vi "Overview.vi"() -> ()   [LabVIEW 2017]
panel:
  out "Time":sgl format="%#_13g"
  out "Flow Rate":sgl caption="C" format="%.1f"
  out "TCHX Power":sgl caption="C" format="%.1f"
  out "DHX Power":dbl caption="C" format="%.1f"
  out "Thermal Power":sgl format="%.1f"
  out "Electrical Power":sgl format="%.1f"
  in  "stop":bool
  out "Fluid Min Temp":sgl format="%.1f"
  out "CTAH Power":sgl format="%.1f"
  out "Fluid Max Temp":sgl format="%.1f"
  out "Heater Power":sgl caption="C" format="%.1f"
  out "LPT Work":sgl format="%.1f"
  out "HPT Work":sgl format="%.1f"
  out "Compressor Work":sgl format="%.1f"
  out "Ambient Temperature":sgl format="%.1f"
  # "Overview"
  # "TCHX"
  # "LPT"
  # "HPT"
  # "COMPRESSOR"
  # "DHX"
  # "CTAH"
  # "HEATER"
  # "PUMP"
  # "NOAH Jr."
  # "Procedures"
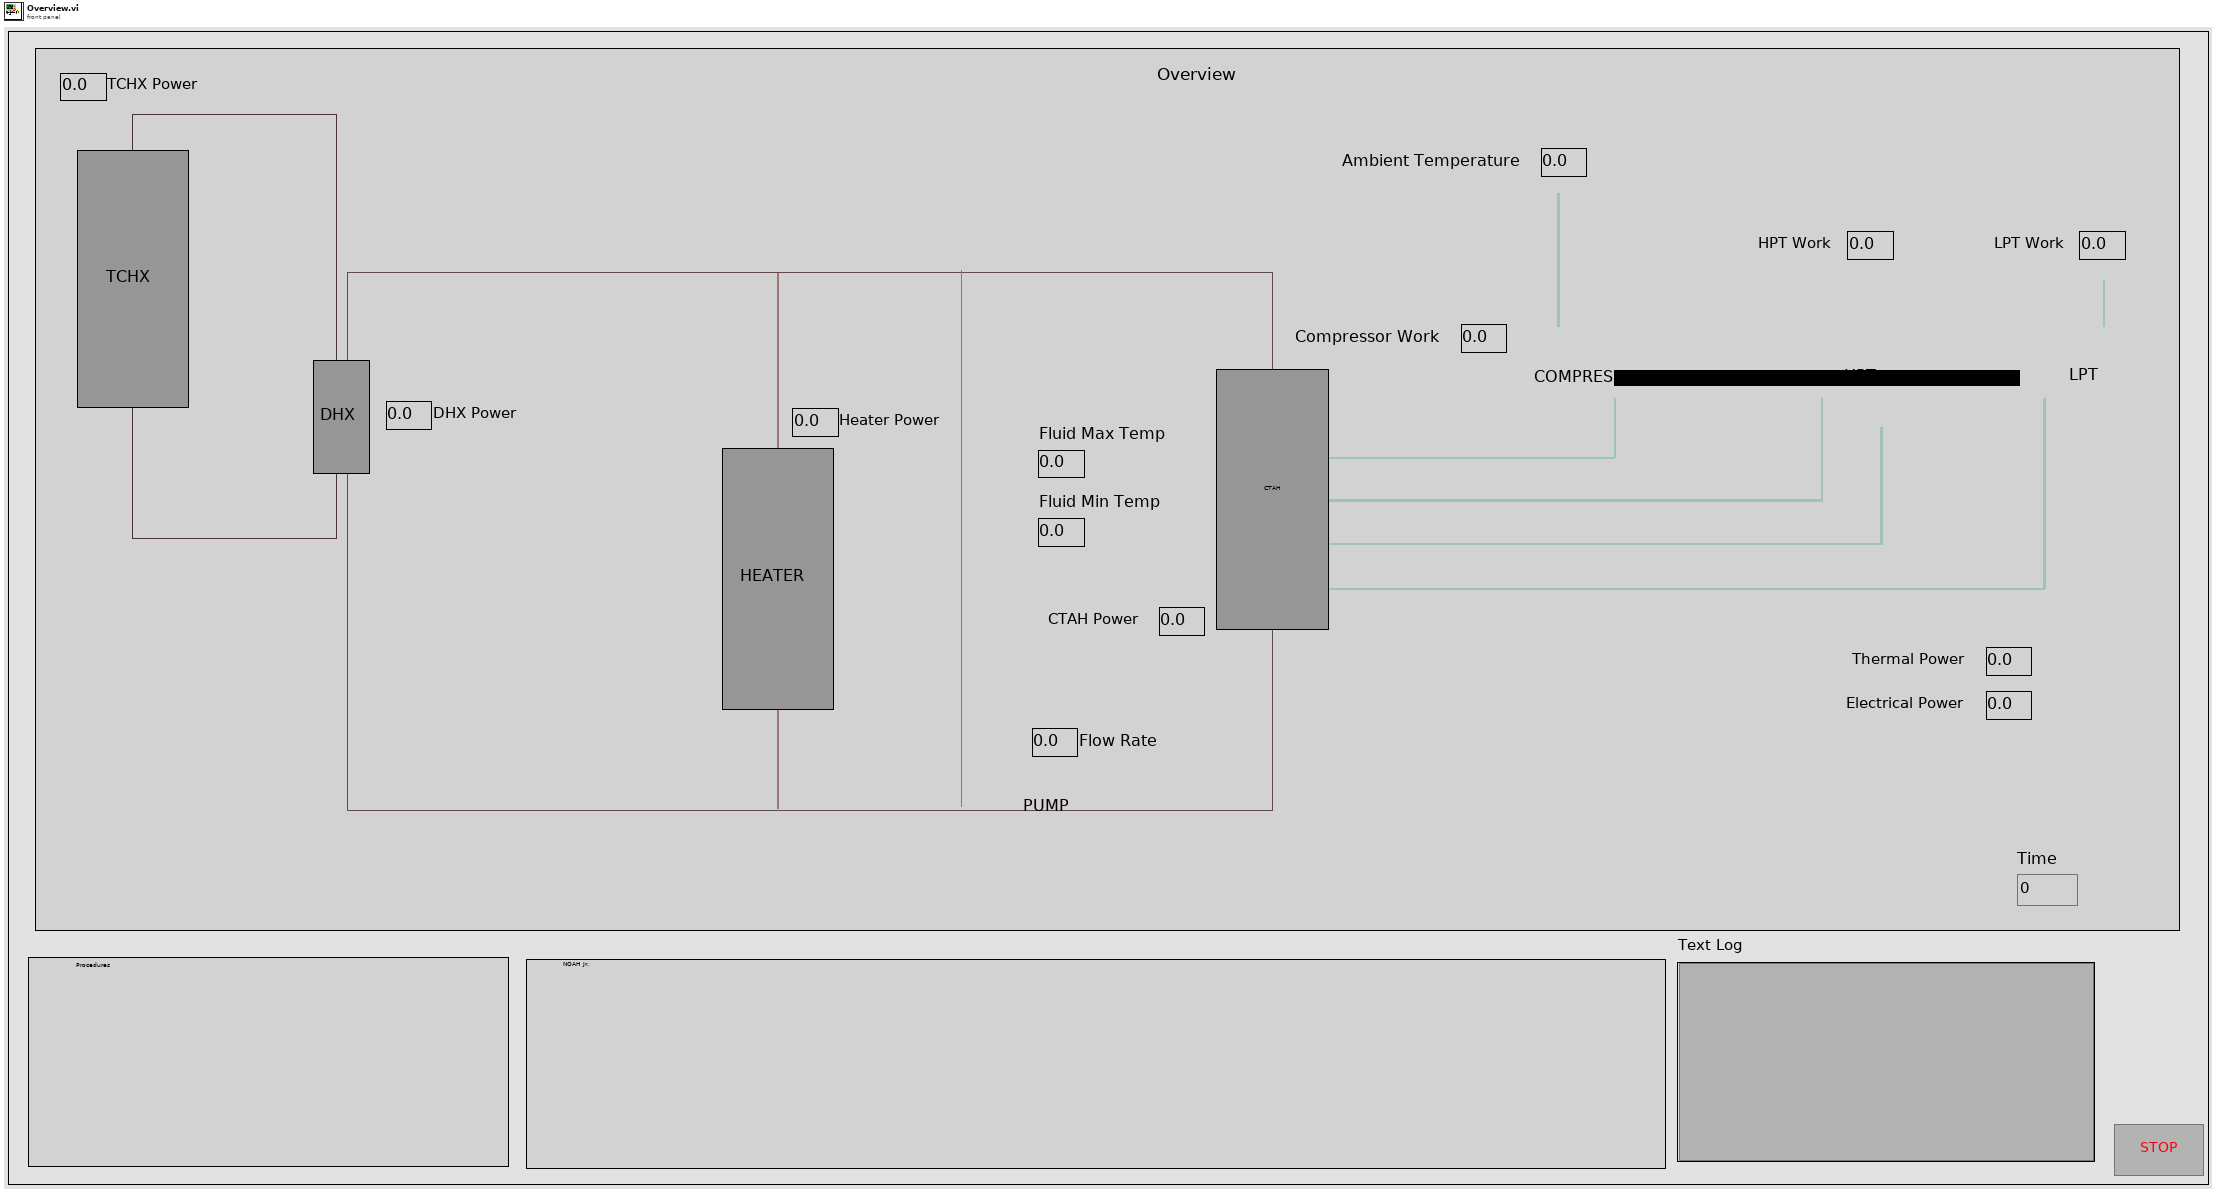
[diagram p1: front panel]
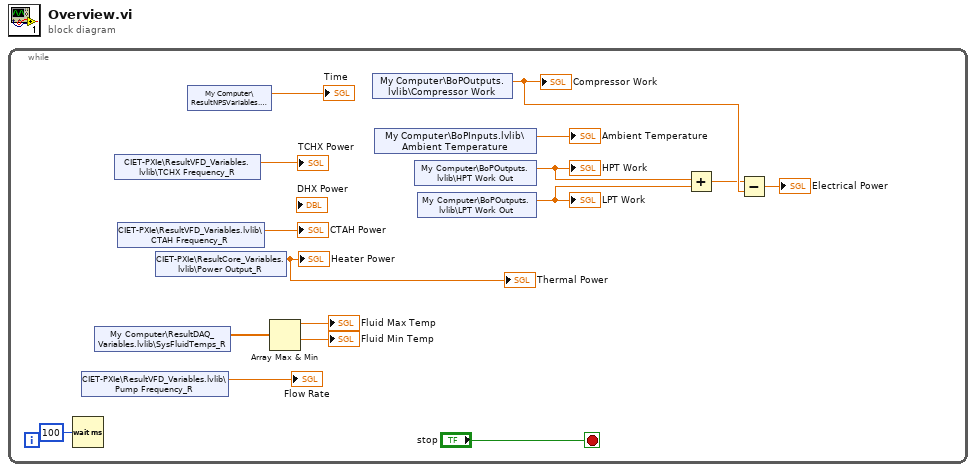
[diagram p0: block diagram]
diagram:
  n1 = while {
    stop <- "stop" stop-if-true
    n2 = Wait (ms)(milliseconds to wait=u32 100) -> ()  [unwired: 1 out]
    n3 = shared-variable "CIET-PXIe\\ResultVFD_Variables.lvlib\\Pump Frequency_R"() -> (→"Flow Rate":sgl)  [unwired: 1 in, 1 out]
    n4 = shared-variable "My Computer\\ResultDAQ_Variables.lvlib\\SysFluidTemps_R"() -> (w13:sgl[])  [unwired: 1 in, 1 out]
    n5 = shared-variable "CIET-PXIe\\ResultVFD_Variables.lvlib\\TCHX Frequency_R"() -> (→"TCHX Power":sgl)  [unwired: 1 in, 1 out]
    n6 = shared-variable "CIET-PXIe\\ResultVFD_Variables.lvlib\\CTAH Frequency_R"() -> (→"CTAH Power":sgl)  [unwired: 1 in, 1 out]
    n7 = shared-variable "CIET-PXIe\\ResultCore_Variables.lvlib\\Power Output_R"() -> (→"Heater Power" →"Thermal Power":sgl)  [unwired: 1 in, 1 out]
    n8 = shared-variable "My Computer\\ResultNPSVariables.lvlib\\Time_R"() -> (→"Time":sgl)  [unwired: 1 in, 1 out]
    n9 = Array Max & Min(array=w13) -> (max value=→"Fluid Max Temp":sgl, min value=→"Fluid Min Temp":sgl)  [unwired: 2 out]
    n10 = shared-variable "My Computer\\BoPOutputs.lvlib\\Compressor Work"() -> (w4:sgl)  [unwired: 1 in, 1 out]
    "Compressor Work" <- w4
    n11 = shared-variable "My Computer\\BoPInputs.lvlib\\Ambient Temperature"() -> (→"Ambient Temperature":sgl)  [unwired: 1 in, 1 out]
    n12 = shared-variable "My Computer\\BoPOutputs.lvlib\\HPT Work Out"() -> (w6:sgl)  [unwired: 1 in, 1 out]
    "HPT Work" <- w6
    n13 = shared-variable "My Computer\\BoPOutputs.lvlib\\LPT Work Out"() -> (w5:sgl)  [unwired: 1 in, 1 out]
    "LPT Work" <- w5
    n14 = Add(x=w6, y=w5) -> (x+y=w3:sgl)
    n15 = Subtract(x=w3, y=w4) -> (x-y=→"Electrical Power":sgl)
  }
